vi "Get System Name.vi"(8 "error in (no error)":errorcluster, 11 "Grabber in":refnum<class "Grabber.lvclass">) -> (0 "error out":errorcluster, 2 "System Name":string, 3 "Grabber out":refnum<class "Grabber.lvclass">)   [LabVIEW 2014, in "Grabber.lvlib" / "Grabber.lvclass"]
uses:
  Grabber.lvclass
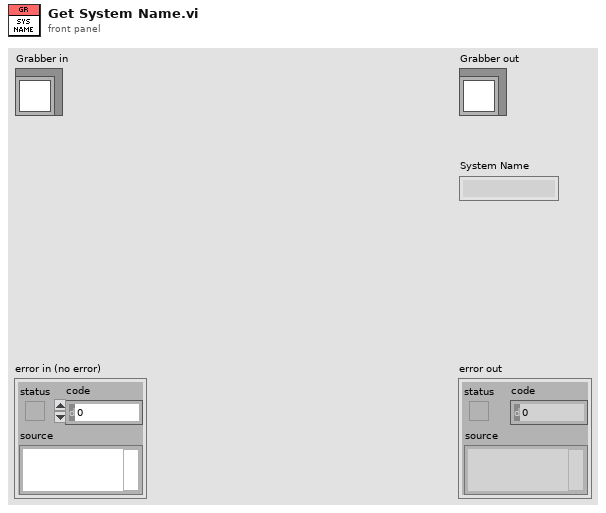
[diagram p1: front panel]
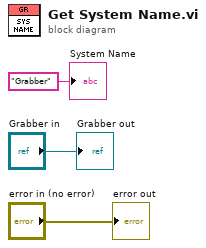
[diagram p0: block diagram]
diagram:
  "error out" <- "error in (no error)"
  "Grabber out" <- "Grabber in"
  "System Name" <- "Grabber"
